vi "Translate Protobuf Error.vi"(8 "error in":errorcluster, 10 "Error Message":string, 11 "Error Code":i32) -> (0 "error out":errorcluster)   [LabVIEW 2019, in "grpc-lvsupport.lvlib"]
uses:
  grpc-lvsupport.lvlib
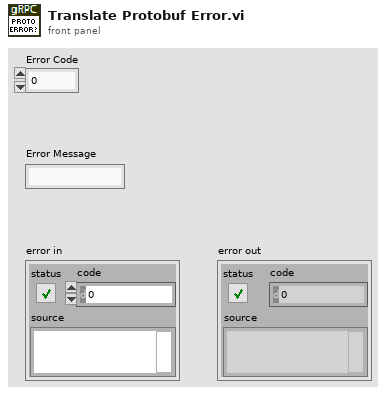
[diagram p1: front panel]
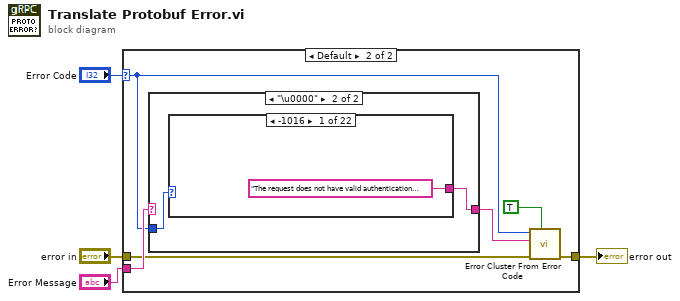
[diagram p0: block diagram]
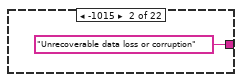
[diagram p4: hidden frame]
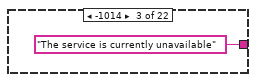
[diagram p5: hidden frame]
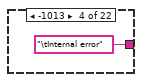
[diagram p6: hidden frame]
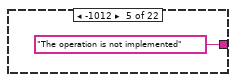
[diagram p7: hidden frame]
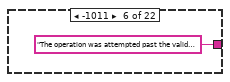
[diagram p8: hidden frame]
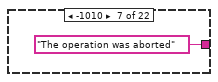
[diagram p9: hidden frame]
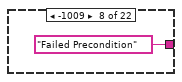
[diagram p10: hidden frame]
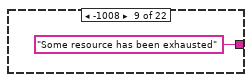
[diagram p11: hidden frame]
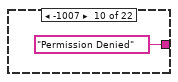
[diagram p12: hidden frame]
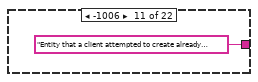
[diagram p13: hidden frame]
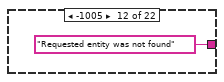
[diagram p14: hidden frame]
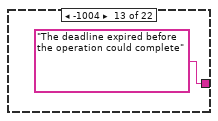
[diagram p15: hidden frame]
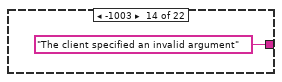
[diagram p16: hidden frame]
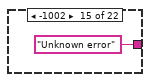
[diagram p17: hidden frame]
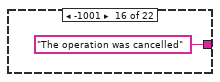
[diagram p18: hidden frame]
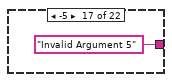
[diagram p19: hidden frame]
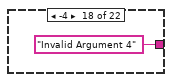
[diagram p20: hidden frame]
diagram:
  n1 = case shown="Default" "Error Code" {
    selector: "Error Code" -> [_ w7]
    tunnel: [w5 w9] -> w1
    tunnel: "Error Message" -> [_ w11]
    tunnel: "error in" -> [w5 w10]
    frame 0 {
    }
    frame Default {
      n2 = case shown="\"\"" w11 {
        selector: w11 -> [w12 _]
        tunnel: w7 -> [_ w14]
        tunnel: [w12 w13] -> w8
        frame Default {
        }
        frame "\u0000" {
          n3 = case shown="-1016" w14 {
            tunnel: ["The request does not have valid authentication credentials" "Unrecoverable data loss or corruption" "The service is currently unavailable" "\tInternal error" "The operation is not implemented" "The operation was attempted past the valid range" "The operation was aborted" "Failed Precondition" "Some resource has been exhausted" "Permission Denied" "Entity that a client attempted to create already exists" "Requested entity was not found" "The deadline expired before the operation could complete" "The client specified an invalid argument" "Unknown error" "The operation was cancelled" "Invalid Argument 5" "Invalid Argument 4" "Invalid Argument 3" "Invalid Argument 2" "Invalid Argument 1" "Unknown Error"] -> w13
            frame -1016 {
            }
            frame -1015 {
            }
            frame -1014 {
            }
            frame -1013 {
            }
            frame -1012 {
            }
            frame -1011 {
            }
            frame -1010 {
            }
            frame -1009 {
            }
            frame -1008 {
            }
            frame -1007 {
            }
            frame -1006 {
            }
            frame -1005 {
            }
            frame -1004 {
            }
            frame -1003 {
            }
            frame -1002 {
            }
            frame -1001 {
            }
            frame -5 {
            }
            frame -4 {
            }
            frame -3 {
            }
            frame -2 {
            }
            frame -1 {
            }
            frame Default {
            }
          }
        }
      }
      n4 = call <vilib>:"Error Cluster From Error Code.vi"("show call chain? (False)"=TRUE ("status"), "error in (no error)"=w10, "error message (\"\")"=w8, "error code (0)"=w7) -> ("error out"=w9:errorcluster)  [unwired: 5 in]
    }
  }
  "error out" <- w1
